vi "Weighted_Cross_Moments.vi"(0 "AI Cluster 1":T3={"Colour"=0, "Inst type"=enum."Pitot-static tube", "Inst name"="Manometer voltage", "Symbol"="U", "Code name"="", "Extra Info"="U", "Inst Array"=enum."PWA", "Extra Titles"=[], "Extra Values"=[], "U"=0.0, "u^2"=0.0, "u^3"=0.0, "u^4"=0.0, "Skew_u"=0.0, "Kurt_u"=0.0, "Sd Error in Mean"=0.0, "% u'/U"=0.0, "X"=0.0, "Y"=0.0, "Z"=0.0, "Timescale integral to 25%"=0.0, "Sd Error in Variance"=0.0, "Calib File"=path "", "Calib Constants"=[], "Output Position"=FALSE, "Full Stats"=FALSE, "Av Sampling Rate"=0.0, "Av No of Samples"=0.0, "Total Meas Time (s)"=0.0, "ADAM Ch Name"=""} {"Sd Error in Variance" format="%.2f"; "Skew_u" format="%.2f"; "% u'/U" format="%.2f"; "Sd Error in Mean" format="%.2f"; "Kurt_u" format="%.2f"; "u^4" format="%.2f"; "u^3" format="%.2f"; "U" format="%.2f"; "u^2" format="%.2f"}, 1 "AI Cluster 2":T3={"Colour"=0, "Inst type"=enum."Pitot-static tube", "Inst name"="Manometer voltage", "Symbol"="U", "Code name"="", "Extra Info"="U", "Inst Array"=enum."PWA", "Extra Titles"=[], "Extra Values"=[], "U"=0.0, "u^2"=0.0, "u^3"=0.0, "u^4"=0.0, "Skew_u"=0.0, "Kurt_u"=0.0, "Sd Error in Mean"=0.0, "% u'/U"=0.0, "X"=0.0, "Y"=0.0, "Z"=0.0, "Timescale integral to 25%"=0.0, "Sd Error in Variance"=0.0, "Calib File"=path "", "Calib Constants"=[], "Output Position"=FALSE, "Full Stats"=FALSE, "Av Sampling Rate"=0.0, "Av No of Samples"=0.0, "Total Meas Time (s)"=0.0, "ADAM Ch Name"=""} {"Sd Error in Variance" format="%.2f"; "Skew_u" format="%.2f"; "% u'/U" format="%.2f"; "Sd Error in Mean" format="%.2f"; "Kurt_u" format="%.2f"; "u^4" format="%.2f"; "u^3" format="%.2f"; "U" format="%.2f"; "u^2" format="%.2f"}, 2 "Time Cluster 1":T1, 3 "Time Cluster 2":T1, 5 "Shift in":dbl[](array[numeric]) format="%.2f") -> (17 "output cluster":T2 {"u^2w^2" format="%.2f"; "u^3w" format="%.2f"; "uw^3" format="%.2f"; "uw/u'w'" format="%.2f"; "uw^2" format="%.2f"; "u^2w" format="%.2f"; "uw" format="%.2f"}, 19 "Shift out":dbl[](array[numeric]) format="%.2f")   [LabVIEW 2013]
uses:
  Controls/Analysis_info_cluster.ctl
  Controls/Inst_type.ctl
  Controls/Instrument_Array.ctl
  Controls/Correlation_cluster1.ctl
  Controls/Time_Trace_Cluster.ctl
  Globals/Meas_global.vi
panel:
  in  "interp. method":i32(ring) items=["nearest", "linear", "spline", "cubic Hermite", "Lagrange"]
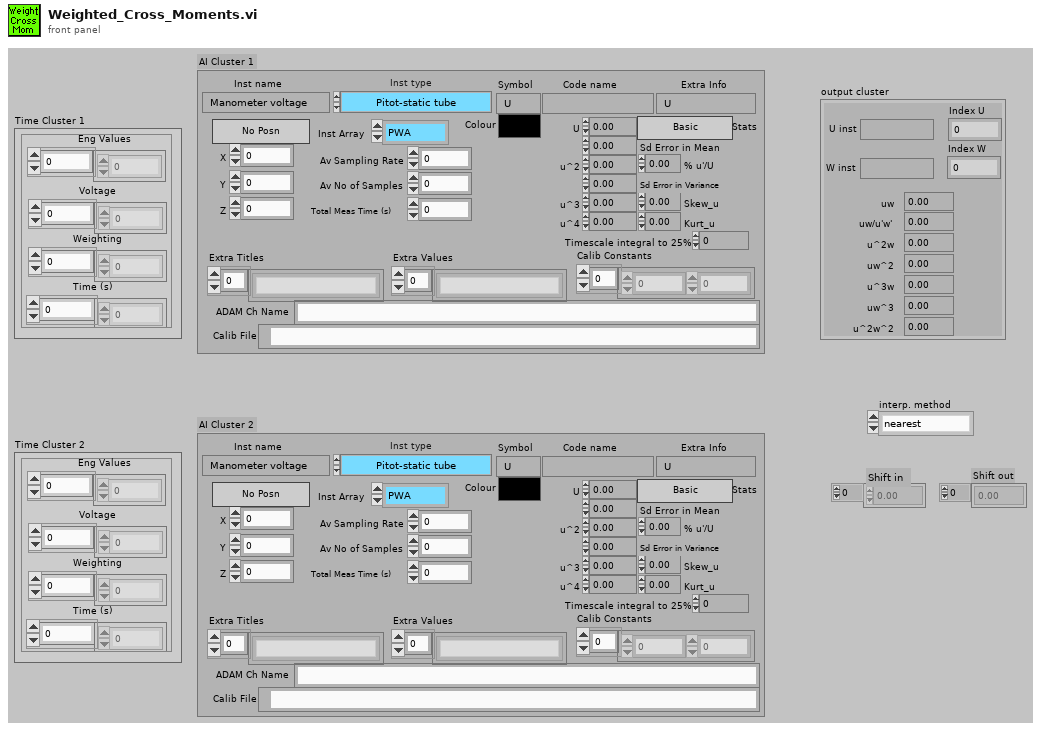
[diagram p1: front panel]
types:
  T1 = typedef "Time_Trace_Cluster.ctl" = cluster{"Weighting":dbl[], "Time (s)":dbl[], "Voltage":dbl[], "Eng Values":dbl[]}
  T2 = typedef "Correlation_cluster1.ctl" = cluster{"U inst":string, "uw":dbl, "u^2w":dbl, "uw^2":dbl, "uw/u'w'":dbl, "W inst":string, "uw^3":dbl, "u^3w":dbl, "u^2w^2":dbl, "Index U":i32, "Index W":i32}
  T3 = typedef "Analysis_info_cluster.ctl" = cluster{"Colour":u32, "Inst type":T4, "Inst name":string, "Symbol":string, "Code name":string, "Extra Info":string, "Inst Array":T5, "Extra Titles":string[], "Extra Values":string[], "U":dbl, "u^2":dbl, "u^3":dbl, "u^4":dbl, "Skew_u":dbl, "Kurt_u":dbl, "Sd Error in Mean":dbl, "% u'/U":dbl, "X":dbl, "Y":dbl, "Z":dbl, "Timescale integral to 25%":dbl, "Sd Error in Variance":dbl, "Calib File":path, "Calib Constants":dbl[], "Output Position":bool, "Full Stats":bool, "Av Sampling Rate":dbl, "Av No of Samples":dbl, "Total Meas Time (s)":dbl, "ADAM Ch Name":string}
  T4 = typedef "Inst_type.ctl" = enum16{"Propeller anemometer", "Raw voltage", "Pressure Transducer", "Pitot-static tube", "Preston tube", "Hot wire", "Cross wire 1", "Cross wire 2", "Generic Linear", "Generic Polynomial", "Generic BackPoly", "Fast FID", "Thermocouple", "Cold wire", "Pulsed Wire", "LDA Vel", "LDA Tran time", "LDA Arr time"}
  T5 = typedef "Instrument_Array.ctl" = enum16{"PWA", "LDA", "Analogue"}
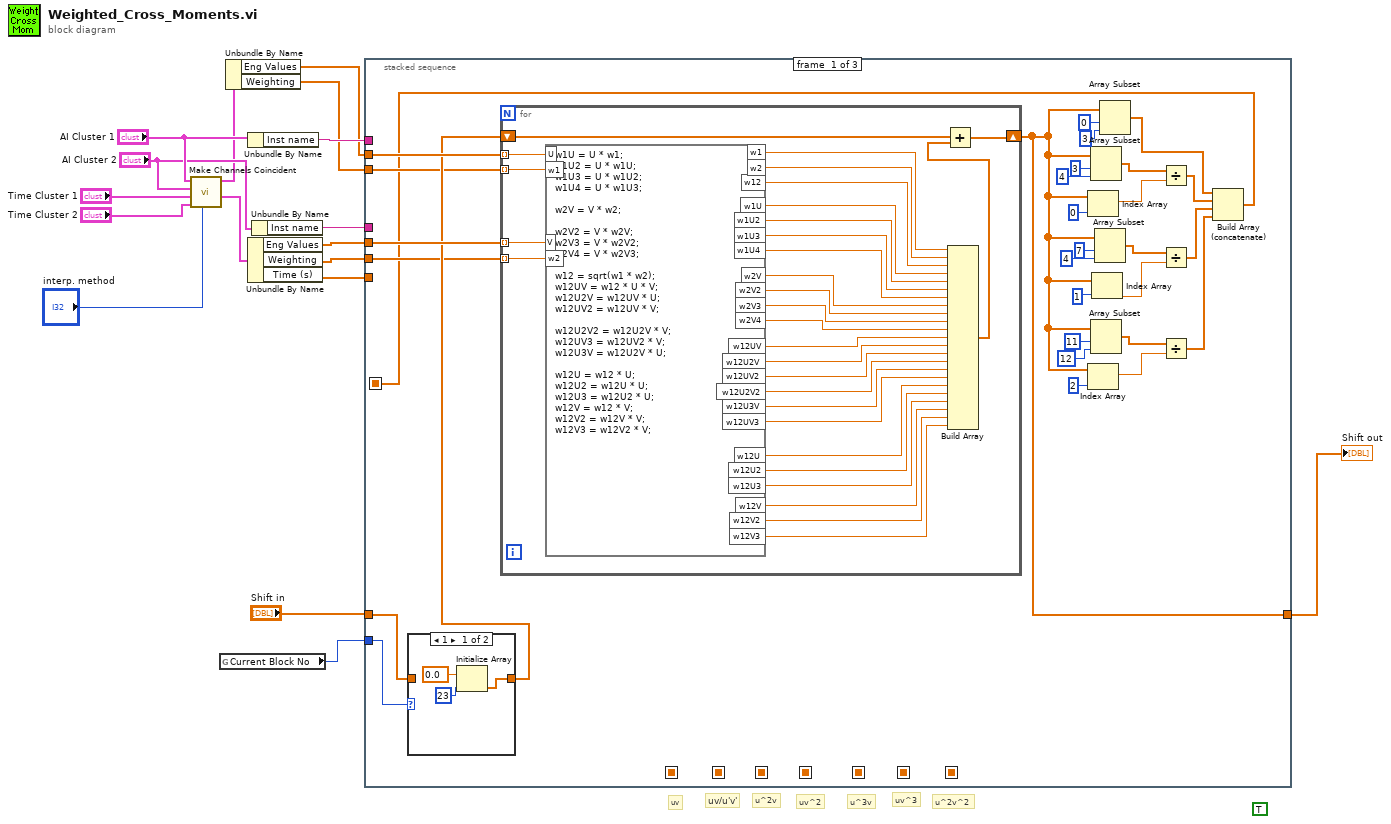
[diagram p0: block diagram]
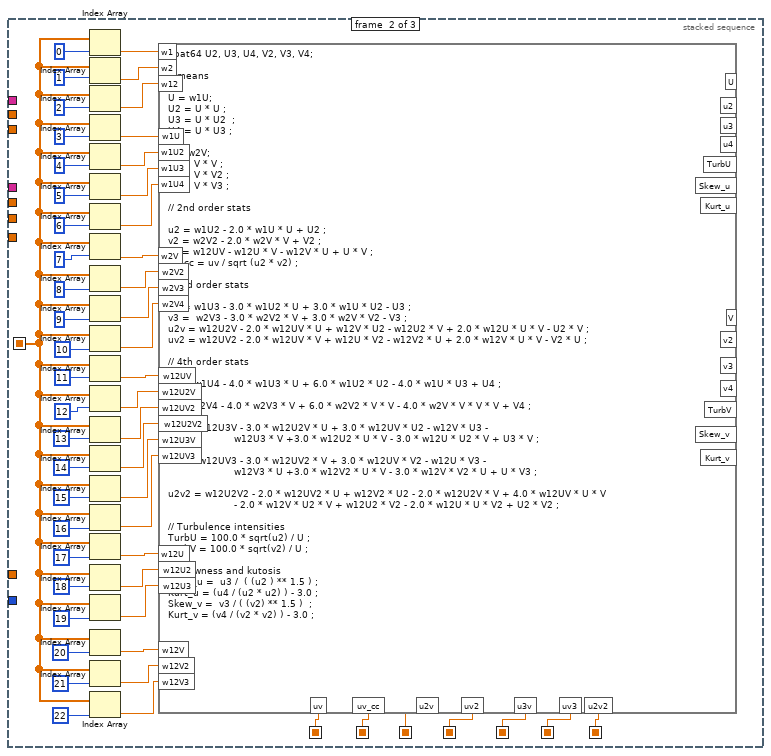
[diagram p3: hidden frame]
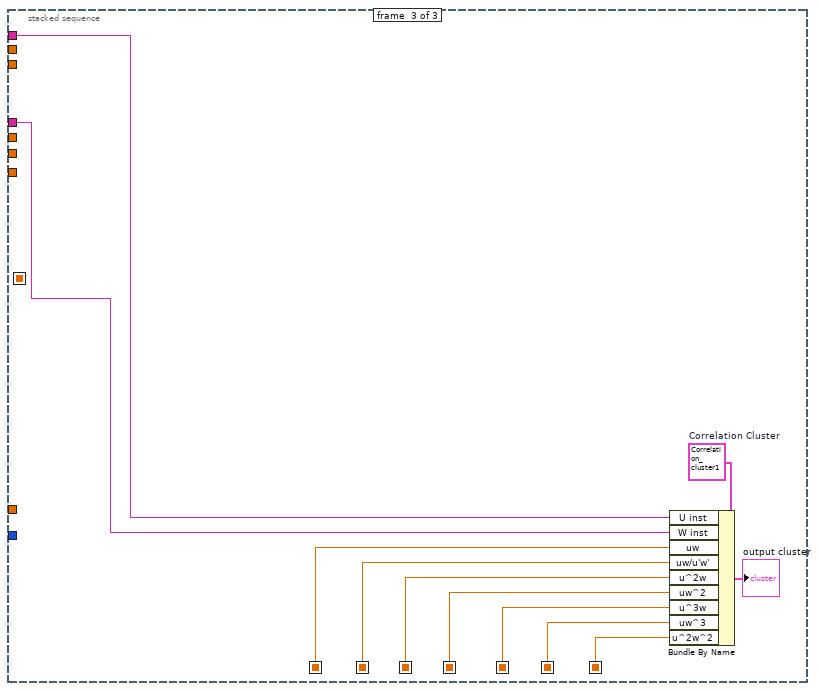
[diagram p4: hidden frame]
diagram:
  (unwired) TRUE
  # "u^2v^2"
  # "uv^3"
  # "u^3v"
  # "uv^2"
  # "u^2v"
  # "uv/u'v'"
  # "uv"
  n1 = call "Make Channels Coincident.vi"("interp. method"="interp. method", "Time Cluster 2"="Time Cluster 2", "Time Cluster 1"="Time Cluster 1", "Cluster 2"="AI Cluster 2", "Cluster 1"="AI Cluster 1") -> ("Coincident Time Cluster 2"=w2:T1, "Coincident Time Cluster 1"=w3:T1)  [unwired: 5 in]
  n2 = global read "Meas_global.vi" "Current Block No"() -> (w15:i32)
  n3 = Unbundle By Name(w3) -> ("Eng Values"=w12:dbl[], "Weighting"=w11:dbl[])
  n4 = Unbundle By Name("AI Cluster 1") -> ("Inst name"=w17:string)
  n5 = Unbundle By Name(w2) -> ("Eng Values"=w10:dbl[], "Weighting"=w9:dbl[], "Time (s)"=w1:dbl[])
  n6 = Unbundle By Name("AI Cluster 2") -> ("Inst name"=w16:string)
  n7 = stacked-sequence {
    seq-local: [_ w123 _] -> [_ _ w143]
    seq-local: [_ w122 _] -> [_ _ w142]
    seq-local: [w40 _ _] -> [_ w84 _]
    seq-local: [_ w117 _] -> [_ _ w141]
    seq-local: [_ w116 _] -> [_ _ w140]
    seq-local: [_ w97 _] -> [_ _ w139]
    seq-local: [_ w96 _] -> [_ _ w138]
    seq-local: [_ w95 _] -> [_ _ w137]
    tunnel: w12 -> [w47 _ _]
    tunnel: "Shift in" -> [w44 _ _]
    tunnel: w10 -> [w46 _ _]
    tunnel: w15 -> [w45 _ _]
    tunnel: w11 -> [w42 _ _]
    tunnel: w9 -> [w41 _ _]
    tunnel: w17 -> [_ _ w145]
    tunnel: w16 -> [_ _ w144]
    tunnel: [w39 _ _] -> w14
    tunnel: w1 -> [_ _ _]
    frame #0 {
      n8 = case shown="1" w45 {
        tunnel: [w48 w51] -> w43
        tunnel: w44 -> [_ w51]
        frame 1 {
          n9 = Initialize Array(0.0 ("Element Data"), 23 ("Dimension Size")) -> (w48:dbl[])
        }
        frame 2, Default {
        }
      }
      n10 = for {
        shift-right: [w77] -> w39
        shift-left: w43 -> [w81]
        tunnel: w42 -> [w76] mode=indexing
        tunnel: w47 -> [w79] mode=indexing
        tunnel: w46 -> [w78] mode=indexing
        tunnel: w41 -> [w75] mode=indexing
        n11 = formula code="w1U = U * w1;\nw1U2 = U * w1U;\nw1U3 = U * w1U2;\nw1U4 = U * w1U3;\n\nw2V = V * w2;\n\nw2V2 = V * w2V;\nw2V3 = V * w2V2;\nw2V4 = V * w2V3;\n\nw12 = sqrt(w1 * w2);\nw12UV = w12 * U * V;\nw12U2V = w12UV * U;\nw12UV2 = w12UV * V;\n\nw12U2V2 = w12U2V * V;\nw12UV3 = w12UV2 * V;\nw12U3V = w12U2V * U;\n\nw12U = w12 * U;\nw12U2 = w12U * U;\nw12U3 = w12U2 * U;\nw12V = w12 * V;\nw12V2 = w12V * V;\nw12V3 = w12V2 * V;"("V"=w78, "U"=w79, "w1"=w76, "w2"=w75) -> ("w12UV"=w66:dbl, "w1U"=w74:dbl, "w2V"=w70:dbl, "w1U2"=w73:dbl, "w2V2"=w69:dbl, "w12U2V"=w65:dbl, "w12UV2"=w64:dbl, "w1U3"=w72:dbl, "w1U4"=w71:dbl, "w2V3"=w68:dbl, "w2V4"=w67:dbl, "w12U3V"=w62:dbl, "w12UV3"=w61:dbl, "w12U2V2"=w63:dbl, "w12U"=w57:dbl, "w12U2"=w56:dbl, "w12U3"=w55:dbl, "w12V"=w54:dbl, "w12V2"=w53:dbl, "w12V3"=w52:dbl, "w12"=w60:dbl, "w1"=w59:dbl, "w2"=w58:dbl)
        n12 = Build Array(w59, w58, w60, w74, w73, w72, w71, w70, w69, w68, w67, w66, w65, w64, w63, w62, w61, w57, w56, w55, w54, w53, w52) -> (w80:dbl[])
        n13 = Add(x=w81, y=w80) -> (x+y=w77:dbl[])
      }
      n14 = Index Array(array=w39, index=0 ("Index")) -> (element=w35:dbl)
      n15 = Index Array(array=w39, index=2 ("Index")) -> (element=w25:dbl)
      n16 = Array Subset(array=w39, index=3 ("Array Index"), length=4) -> (w36:dbl[])
      n17 = Array Subset(array=w39, index=11 ("Array Index"), length=12) -> (w26:dbl[])
      n18 = Index Array(array=w39, index=1 ("Index")) -> (element=w32:dbl)
      n19 = Array Subset(array=w39, index=7 ("Array Index"), length=4) -> (w31:dbl[])
      n20 = Array Subset(array=w39, index=0, length=3) -> (w18:dbl[])
      n21 = Divide(x=w36, y=w35) -> (x/y=w23:dbl[])
      n22 = Divide(x=w31, y=w32) -> (x/y=w22:dbl[])
      n23 = Divide(x=w26, y=w25) -> (x/y=w21:dbl[])
      n24 = Build Array (concatenate)(w18, w23, w22, w21) -> (w40:dbl[])
    }
    frame #1 {
      n25 = Index Array(array=w84, index=0) -> (element=w129:dbl)
      n26 = Index Array(array=w84, index=1) -> (element=w128:dbl)
      n27 = Index Array(array=w84, index=2) -> (element=w127:dbl)
      n28 = Index Array(array=w84, index=3) -> (element=w126:dbl)
      n29 = Index Array(array=w84, index=4) -> (element=w125:dbl)
      n30 = Index Array(array=w84, index=5) -> (element=w124:dbl)
      n31 = Index Array(array=w84, index=6) -> (element=w119:dbl)
      n32 = Index Array(array=w84, index=7) -> (element=w118:dbl)
      n33 = Index Array(array=w84, index=8) -> (element=w109:dbl)
      n34 = Index Array(array=w84, index=9) -> (element=w108:dbl)
      n35 = Index Array(array=w84, index=10) -> (element=w111:dbl)
      n36 = Index Array(array=w84, index=11) -> (element=w110:dbl)
      n37 = Index Array(array=w84, index=12) -> (element=w105:dbl)
      n38 = Index Array(array=w84, index=13) -> (element=w104:dbl)
      n39 = Index Array(array=w84, index=14) -> (element=w100:dbl)
      n40 = Index Array(array=w84, index=15) -> (element=w99:dbl)
      n41 = Index Array(array=w84, index=16) -> (element=w98:dbl)
      n42 = Index Array(array=w84, index=17) -> (element=w90:dbl)
      n43 = Index Array(array=w84, index=18) -> (element=w89:dbl)
      n44 = Index Array(array=w84, index=19) -> (element=w88:dbl)
      n45 = Index Array(array=w84, index=20) -> (element=w87:dbl)
      n46 = Index Array(array=w84, index=21) -> (element=w83:dbl)
      n47 = Index Array(array=w84, index=22) -> (element=w82:dbl)
      n48 = formula code="float64 U2, U3, U4, V2, V3, V4;\n\n// means\n\nU = w1U;\nU2 = U * U ;\nU3 = U * U2  ;\nU4 = U * U3 ;\n\nV = w2V;\nV2 = V * V ;\nV3 = V * V2 ;\nV4 = V * V3 ;\n\n// 2nd order stats\n\nu2 = w1U2 - 2.0 * w1U * U + U2 ;\nv2 = w2V2 - 2.0 * w2V * V + V2 ;\nuv = w12UV - w12U * V - w12V * U + U * V ;\nuv_cc = uv / sqrt (u2 * v2) ;\n\n// 3rd order stats\n\nu3 = w1U3 - 3.0 * w1U2 * U + 3.0 * w1U * U2 - U3 ;\nv3 =  w2V3 - 3.0 * w2V2 * V + 3.0 * w2V * V2 - V3 ;\nu2v = w12U2V - 2.0 * w12UV * U + w12V * U2 - w12U2 * V + 2.0 * w12U * U * V - U2 * V ;\nuv2 = w12UV2 - 2.0 * w12UV * V + w12U * V2 - w12V2 * U + 2.0 * w12V * U * V - V2 * U ;\n\n// 4th order stats\n\nu4 = w1U4 - 4.0 * w1U3 * U + 6.0 * w1U2 * U2 - 4.0 * w1U * U3 + U4 ;\n\nv4 = w2V4 - 4.0 * w2V3 * V + 6.0 * w2V2 * V * V - 4.0 * w2V * V * V * V + V4 ;\n\nu3v = w12U3V - 3.0 * w12U2V * U + 3.0 * w12UV * U2 - w12V * U3 - \n                      w12U3 * V +3.0 * w12U2 * U * V - 3.0 * w12U * U2 * V + U3 * V ;\n\nuv3 = w12UV3 - 3.0 * w12UV2 * V + 3.0 * w12UV * V2 - w12U * V3 - \n                      w12V3 * U +3.0 * w12V2 * U * V - 3.0 * w12V * V2 * U + U * V3 ;\n\nu2v2 = w12U2V2 - 2.0 * w12UV2 * U + w12V2 * U2 - 2.0 * w12U2V * V + 4.0 * w12UV * U * V\n                      - 2.0 * w12V * U2 * V + w12U2 * V2 - 2.0 * w12U * U * V2 + U2 * V2 ; \n\n// Turbulence intensities\nTurbU = 100.0 * sqrt(u2) / U ;\nTurbV = 100.0 * sqrt(v2) / U ;\n\n// Skewness and kutosis\nSkew_u =  u3 /  ( (u2 ) ** 1.5 ) ;\nKurt_u = (u4 / (u2 * u2) ) - 3.0 ;\nSkew_v =  v3 / ( (v2) ** 1.5 )  ;\nKurt_v = (v4 / (v2 * v2) ) - 3.0 ;"("w1"=w129, "w2"=w128, "w12"=w127, "w1U2"=w125, "w1U3"=w124, "w1U"=w126, "w1U4"=w119, "w2V"=w118, "w2V2"=w109, "w2V4"=w111, "w2V3"=w108, "w12UV"=w110, "w12U2V"=w105, "w12UV2"=w104, "w12U2V2"=w100, "w12U3V"=w99, "w12UV3"=w98, "w12U2"=w89, "w12U3"=w88, "w12V"=w87, "w12V2"=w83, "w12U"=w90, "w12V3"=w82) -> ("uv"=w123:dbl, "uv_cc"=w122:dbl, "u2v"=w117:dbl, "uv2"=w116:dbl, "u3v"=w97:dbl, "uv3"=w96:dbl, "u2v2"=w95:dbl)  [unwired: 14 out]
    }
    frame #2 {
      w146 = T2 {"U inst"="", "uw"=0.0, "u^2w"=0.0, "uw^2"=0.0, "uw/u'w'"=0.0, "W inst"="", "uw^3"=0.0, "u^3w"=0.0, "u^2w^2"=0.0, "Index U"=0, "Index W"=0}  # Correlation Cluster
      n49 = Bundle By Name(cluster=w146, "U inst"=w145, "W inst"=w144, "uw"=w143, "uw/u'w'"=w142, "u^2w"=w141, "uw^2"=w140, "u^3w"=w139, "uw^3"=w138, "u^2w^2"=w137) -> (→"output cluster":T2)
    }
  }
  "Shift out" <- w14
